vi "Init.vi"(6 "Creator":refnum<class "Msg Type Strategy.lvclass">, 8 "Creator Alias":string, 9 "Self":refnum<class "Msg Type Strategy.lvclass">, 10 "Self Alias":string) -> (3 "Addresses out":refnum<class "Addresses.lvclass">)   [LabVIEW 2021, in "jettl.lvlib" / "Addresses.lvlib" / "Addresses.lvclass"]
uses:
  Addresses.lvclass
  Msg Type Strategy/Msg Type Strategy/Msg Type Strategy.lvclass
  Created.ctl
  Addresses.lvclass/Addresses.ctl
  Addresses.lvlib
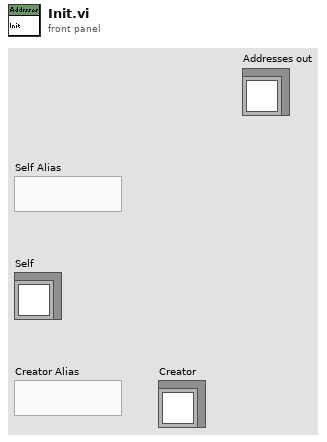
[diagram p1: front panel]
types:
  T1 = typedef "jettl.lvlib/Addresses.lvlib/Created.ctl" = map{string, refnum<class "Msg Type Strategy.lvclass">}
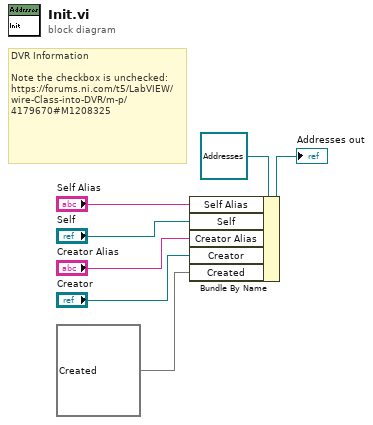
[diagram p0: block diagram]
diagram:
  # "DVR Information\n\nNote the checkbox is unchecked:\nhttps://forums.ni.com/t5/LabVIEW/wire-Class-into-DVR/m-p/4179670#M1208325"
  n1 = Bundle By Name(cluster=refnum<class "Addresses.lvclass"> refnum ("Queue Mailbox out"), "Self Alias"="Self Alias", "Self"="Self", "Creator Alias"="Creator Alias", "Creator"="Creator", "Created"=T1 {}) -> (→"Addresses out":refnum<class "Addresses.lvclass">)
